vi "Process.vi"(0 "Module Data In":T1, 11 "error in (no error)":errorcluster) -> (4 "Module Data Out":T1, 15 "error out":errorcluster)   [LabVIEW 2017, in "Error Handler - Logger.lvlib"]
doc: "Initializes and run the processes in the Process Array one after the other."
uses:
  Error Handler - Logger.lvlib
  Controls/Module - Data.ctl
  Modules.ctl
  Controls/Module - States.ctl
  Controls/Timing - Data.ctl
  Controls/Process - Element.ctl
  Controls/Process.ctl
  Controls/Process - Status.ctl
  Controls/Current Error Details.ctl
  Controls/Error Types.ctl
panel:
  in  "Process Status":string
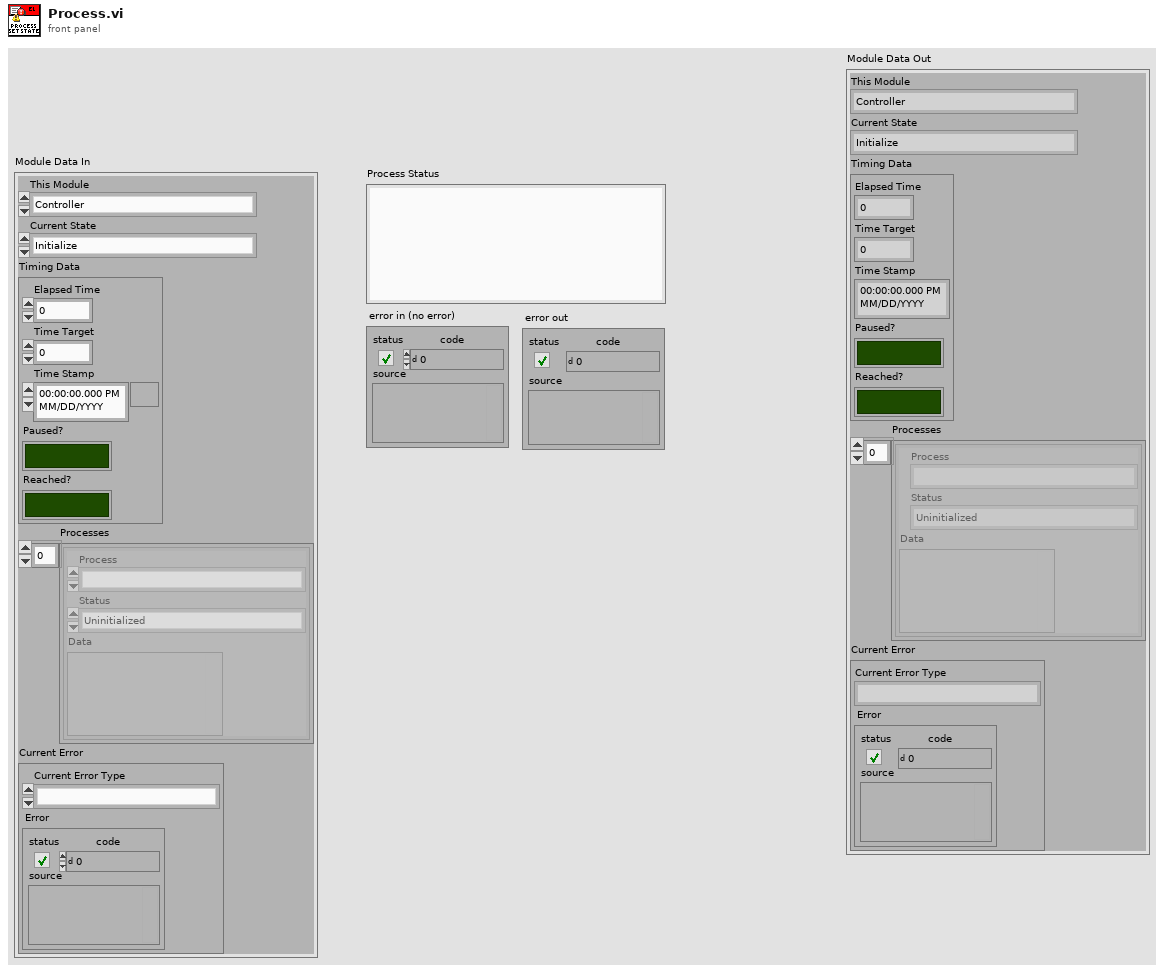
[diagram p1: front panel]
types:
  T1 = typedef "Error Handler - Logger.lvlib/Module - Data.ctl" = cluster{"This Module":T2, "Current State":T3, "Timing Data":T4, "Processes":T5[], "Current Error":T8}
  T2 = typedef "Error Handler - Logger.lvlib/Modules.ctl" = enum16{"Controller", "Error Handler - Logger"}
  T3 = typedef "Error Handler - Logger.lvlib/Module - States.ctl" = enum16{"Initialize", "Event ", "Send data", "FP Element: Update", "FP Element: Disable/Enable", "Timer: Setup", "Terminate", "--------Template----------", "Process Error", "Log ", "Log Error"}
  T4 = typedef "Error Handler - Logger.lvlib/Timing - Data.ctl" = cluster{"Elapsed Time":dbl, "Time Target":dbl, "Time Stamp":timestamp, "Paused?":bool, "Reached?":bool}
  T5 = typedef "Error Handler - Logger.lvlib/Process - Element.ctl" = cluster{"Process":T6, "Status":T7, "Data":variant}
  T6 = typedef "Error Handler - Logger.lvlib/Process.ctl" = enum16{""}
  T7 = typedef "Error Handler - Logger.lvlib/Process - Status.ctl" = enum16{"Uninitialized", "Busy"}
  T8 = typedef "Error Handler - Logger.lvlib/Current Error Details.ctl" = cluster{"Current Error Type":T9, "Error":errorcluster}
  T9 = typedef "Error Handler - Logger.lvlib/Error Types.ctl" = enum16{""}
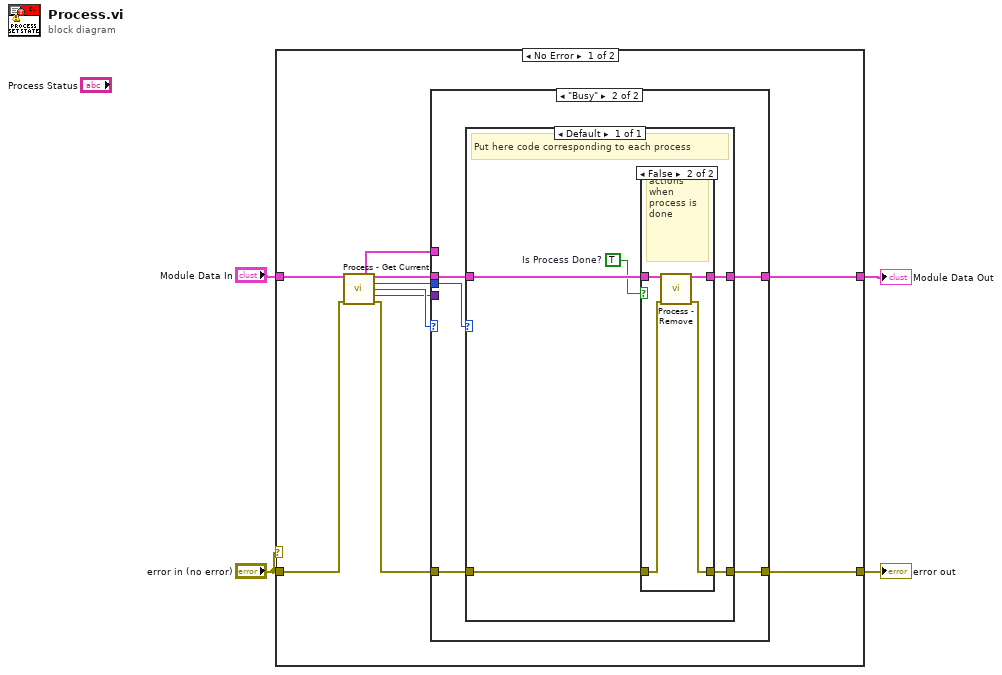
[diagram p0: block diagram]
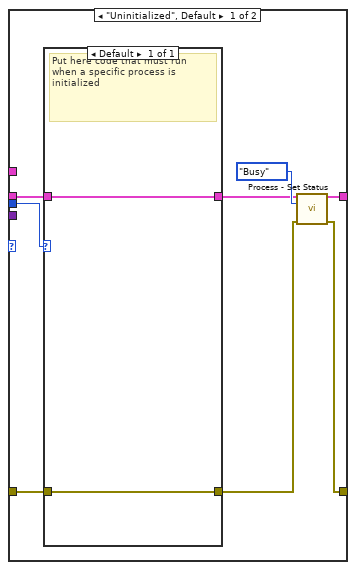
[diagram p2: hidden frame]
diagram:
  n1 = case shown="No Error" "error in (no error)" {
    tunnel: [w13 w42] -> w4
    tunnel: "Module Data In" -> [w14 w42]
    tunnel: [w11 w41] -> w2
    tunnel: "error in (no error)" -> [w6 w41]
    frame No Error {
      n2 = call "Process - Get Current.vi"("Module Data In"=w14, "error in (no error)"=w6) -> ("|Current Process"=w7:T5, "Module Data Out"=w12:T1, "Process"=w10:T6, "Status"=w9:T7, "Data"=w8:variant, "error out"=w5:errorcluster)  [unwired: 8 in]
      n3 = case shown="\"Busy\"" w9 {
        tunnel: [w22 w28] -> w13
        tunnel: w12 -> [w20 w29]
        tunnel: [w15 w25] -> w11
        tunnel: w5 -> [w18 w27]
        tunnel: w10 -> [w17 w26]
        tunnel: w8 -> [_ _]
        tunnel: w7 -> [_ _]
        frame "Uninitialized", Default {
          n4 = case shown="Default" w17 {
            tunnel: [w23] -> w19
            tunnel: w20 -> [w23]
            tunnel: [w24] -> w16
            tunnel: w18 -> [w24]
            frame Default {
              # "Put here code that must run when a specific process is initialized"
            }
          }
          n5 = call "Process - Set Status.vi"("Module Data In"=w19, "Status"=Process_-_Status."Busy", "error in (no error)"=w16) -> ("Module Data Out"=w22:T1, "error out"=w15:errorcluster)  [unwired: 11 in]
        }
        frame "Busy" {
          n6 = case shown="Default" w26 {
            tunnel: [w33] -> w28
            tunnel: w29 -> [w34]
            tunnel: [w31] -> w25
            tunnel: w27 -> [w32]
            frame Default {
              w30 = TRUE  # Is Process Done?
              # "Put here code corresponding to each process"
              n7 = case shown="False" w30 {
                tunnel: [w35 w39] -> w33
                tunnel: w34 -> [w35 w40]
                tunnel: [w36 w37] -> w31
                tunnel: w32 -> [w36 w38]
                frame True {
                  # "Actions while process is still running"
                }
                frame False {
                  # "actions\nwhen process is done"
                  n8 = call "Process - Remove.vi"("Module Data In"=w40, "error in (no error)"=w38) -> ("Module Data Out"=w39:T1, "error out"=w37:errorcluster)  [unwired: 12 in]
                }
              }
            }
          }
        }
      }
    }
    frame Error {
    }
  }
  "error out" <- w2
  "Module Data Out" <- w4
